vi "Read Session Information.vi"(8 "error in (no error)":errorcluster, 11 "TwinCAT ADS in":refnum<class "TwinCAT ADS.lvclass">) -> (0 "error out":errorcluster, 1 "Session Infomation":T1, 3 "TwinCAT ADS out":refnum<class "TwinCAT ADS.lvclass">)   [LabVIEW 2018, in "TwinCAT ADS.lvclass"]
uses:
  TwinCAT ADS.lvclass
  Controls/Session Information.ctl
  Controls/Connection State.ctl
  TwinCAT ADS.lvclass/TwinCAT ADS.ctl
  TwinCAT.Ads
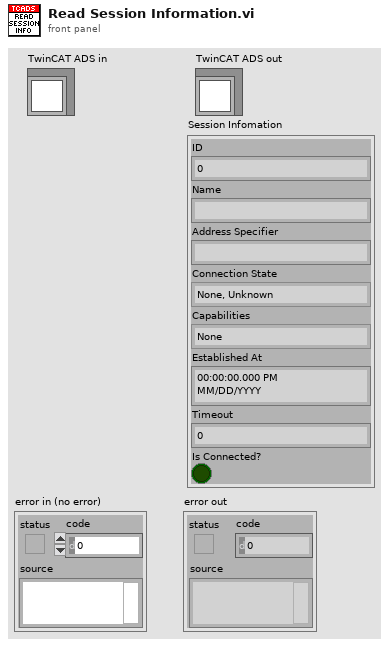
[diagram p1: front panel]
types:
  T1 = typedef "TwinCAT ADS.lvclass/Session Information.ctl" = cluster{"ID":i32, "Name":string, "Address Specifier":string, "Connection State":T2, "Capabilities":enum16{"None", "DataTypeSupport", "SymbolBrowsing", "ValueRead", "ValueWrite", "ValueNotifications", "Mask_All"}, "Established At":timestamp, "Timeout":i32, "Is Connected?":bool}
  T2 = typedef "TwinCAT ADS.lvclass/Connection State.ctl" = enum16{"None, Unknown", "Disconnected", "Connected", "Lost"}
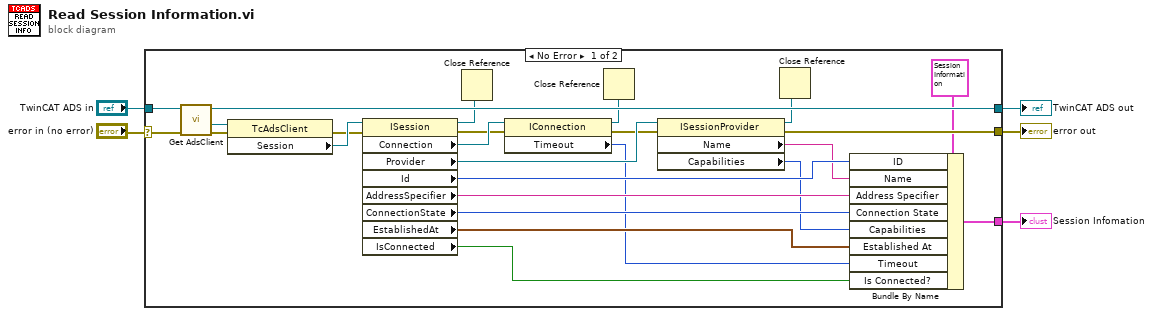
[diagram p0: block diagram]
diagram:
  n1 = case shown="No Error" "error in (no error)" {
    selector: "error in (no error)" -> [w13 w32]
    tunnel: [w18 w32] -> w4
    tunnel: [w11 w31] -> w2
    tunnel: "TwinCAT ADS in" -> [w12 w31]
    tunnel: [w17 _] -> w1
    frame No Error {
      n2 = call "Get AdsClient.vi"("error in (no error)"=w13, "TwinCAT ADS in"=w12) -> ("error out"=w15:errorcluster, ".NET TcAdsClient"=w14:refnum<k24>, "TwinCAT ADS out"=w11:refnum<class "TwinCAT ADS.lvclass">)  [unwired: 7 in]
      n3 = property class="TcAdsClient"(reference=w14, error in=w15) -> (error out=w29:errorcluster, "Session"=w30:refnum<k24>)  [unwired: 1 out]
      n4 = property class="ISession"(reference=w30, error in=w29) -> (reference out=w8:refnum<k24>, error out=w9:errorcluster, "Connection"=w16:refnum<k24>, "Provider"=w28:refnum<k24>, "Id"=w26:i32, "AddressSpecifier"=w24:string, "ConnectionState"=w23:i32, "EstablishedAt"=w21:timestamp, "IsConnected"=w19:bool)
      n5 = Close Reference(reference=w8) -> ()  [unwired: 1 in, 1 out]
      n6 = property class="IConnection"(reference=w16, error in=w9) -> (reference out=w7:refnum<k24>, error out=w27:errorcluster, "Timeout"=w20:i32)
      n7 = Close Reference(reference=w7) -> ()  [unwired: 1 in, 1 out]
      n8 = property class="ISessionProvider"(reference=w28, error in=w27) -> (reference out=w6:refnum<k24>, error out=w18:errorcluster, "Name"=w25:string, "Capabilities"=w22:i32)
      n9 = Close Reference(reference=w6) -> ()  [unwired: 1 in, 1 out]
      n10 = Bundle By Name(cluster=T1 {"ID"=0, "Name"="", "Address Specifier"="", "Connection State"=enum."None, Unknown", "Capabilities"=enum."None", "Established At"=timestamp(0 s since 1904-01-01), "Timeout"=0, "Is Connected?"=FALSE} ("Session Infomation"), "ID"=w26, "Name"=w25, "Address Specifier"=w24, "Connection State"=w23, "Capabilities"=w22, "Established At"=w21, "Timeout"=w20, "Is Connected?"=w19) -> (w17:T1)
    }
    frame Error {
    }
  }
  "error out" <- w4
  "TwinCAT ADS out" <- w2
  "Session Infomation" <- w1
